vi "Get TC Reference.vi"(8 "error in (no error)":errorcluster, 11 "VISA resource name":refnum<visa-resource-name>) -> (0 "error out":errorcluster, 1 "External Reference Value":dbl format="%.4f", 2 "Reference Source":u16, 3 "VISA resource name out":refnum<visa-resource-name>, 4 "Temperature Units":i32)   [LabVIEW 2011, in "Fluke 5XXX Series Multicalibrators.lvlib"]
doc: "This VI returns the source and value of the temperature being used as a reference for thermocouple simulation and measurement (in Celsius, CEL, or Fahrenheit, FAR, depending on active units).\n\nNote:\n\nThis VI is available only for instrument models 5500A and 5520A."
uses:
  Fluke 5XXX Series Multicalibrators.lvlib
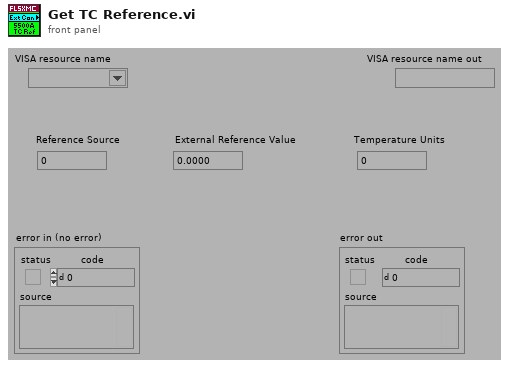
[diagram p1: front panel]
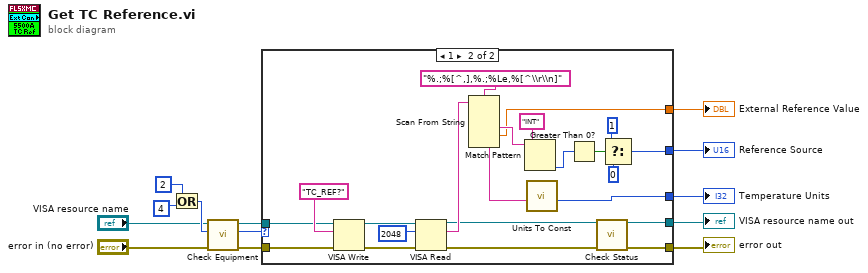
[diagram p0: block diagram]
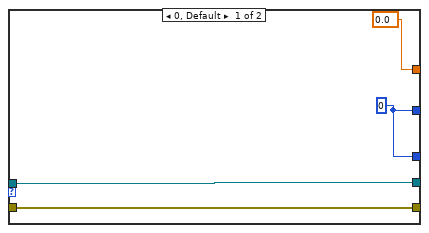
[diagram p2: hidden frame]
diagram:
  n1 = Or(x=2 ("Numeric"), y=4 ("Numeric")) -> (x .or. y?=w8:i32)
  n2 = call "Check Equipment.vi"("error in (no error)"="error in (no error)", "Bit Mask"=w8, "VISA resource name"="VISA resource name") -> ("error out"=w13:errorcluster, "Present?"=w12:u32, "VISA resource name out"=w11:refnum<visa-resource-name>)  [unwired: 6 in]
  n3 = case shown="1" w12 {
    tunnel: [w17 w33] -> w5
    tunnel: [w16 w32] -> w4
    tunnel: w13 -> [w17 w35]
    tunnel: w11 -> [w16 w34]
    tunnel: [w14 w23] -> w3
    tunnel: [0.0 w22] -> w2
    tunnel: [w14 w21] -> w1
    frame 0, Default {
      w14 = u16 0
    }
    frame 1 {
      n4 = VISA Write(VISA resource name=w34, write buffer="TC_REF?", error in (no error)=w35) -> (VISA resource name out=w38:refnum<visa-resource-name>, error out=w37:errorcluster)  [unwired: 1 out]
      n5 = VISA Read(VISA resource name=w38, byte count=u32 2048 ("byte count (0)"), error in (no error)=w37) -> (VISA resource name out=w19:refnum<visa-resource-name>, read buffer=w25:string, error out=w20:errorcluster)  [unwired: 1 out]
      n6 = Scan From String(format string="%.;%[^,],%.;%Le,%[^\\r\\n]", input string=w25) -> (output 1=w24:string, output 2=w22:dbl, output 3=w18:string)  [unwired: 5 in, 3 out]
      n7 = Match Pattern(string=w24, regular expression="INT") -> (offset past match=w29:i32)  [unwired: 1 in, 3 out]
      n8 = call "Units To Const.vi"("Units"=w18) -> ("Const"=w21:i32)  [unwired: 10 in]
      n9 = Greater Than 0?(x=w29) -> (x > 0?=w26:bool)
      n10 = call "Check Status.vi"("VISA resource name"=w19, "error in (no error)"=w20) -> ("VISA resource name out"=w32:refnum<visa-resource-name>, "error out"=w33:errorcluster)  [unwired: 12 in]
      n11 = Select(t=u16 1 ("f"), s=w26, f=u16 0) -> (s? t:f=w23:u16)
    }
  }
  "Reference Source" <- w3
  "External Reference Value" <- w2
  "Temperature Units" <- w1
  "VISA resource name out" <- w4
  "error out" <- w5
